vi "Get Instance Lookup.vi"(8 "error in (no error)":errorcluster, 10 "Create If Not Exist (T)":bool=TRUE, 11 "WebSocket In":refnum<class "Websocket.lvclass">) -> (0 "error out":errorcluster, 1 "NewObjectCreated":bool, 2 "DVRRefOut":refnum<data-value>, 3 "WebSocket Out":refnum<class "Websocket.lvclass">, 5 "ObjectQueueName":string caption="This queue name could be used to destroy\nthe named queue that is used to hold the\nreference in the clean up.")   [LabVIEW 2015]
uses:
  Websocket.lvclass
  Object Attributes.ctl
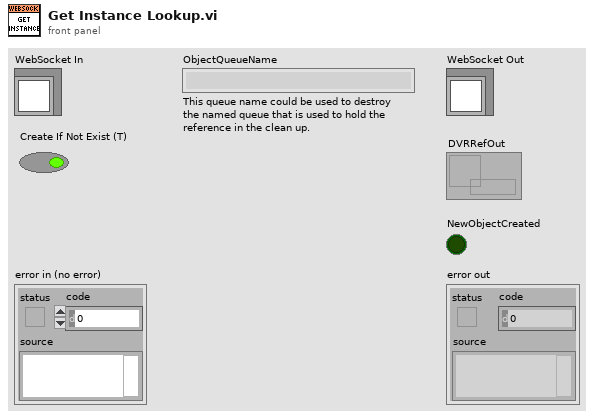
[diagram p1: front panel]
types:
  T1 = enum16{"Create or look up existing", "Look up existing"}
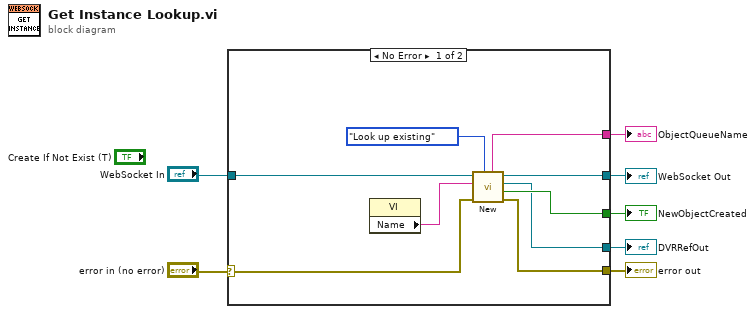
[diagram p0: block diagram]
diagram:
  n1 = case shown="No Error" "error in (no error)" {
    selector: "error in (no error)" -> [w15 w18]
    tunnel: [w16 w17] -> w7
    tunnel: [w14 w18] -> w5
    tunnel: "WebSocket In" -> [w12 w17]
    tunnel: [w11 _] -> w3
    tunnel: [w10 _] -> w2
    tunnel: [w8 _] -> w1
    frame No Error {
      n2 = property class="VI"() -> ("Name"=w13:string)  [unwired: 2 in, 2 out]
      n3 = call "New.vi"("CreateMethod(Create or look up existing)"=T1."Look up existing", "error in (no error)"=w15, "Object name"=w13, "Websocket In"=w12) -> ("error out"=w14:errorcluster, "NewObjectCreated"=w11:bool, "DVRRefOut"=w10:refnum<data-value>, "Websocket Out"=w16:refnum<class "Websocket.lvclass">, "ObjectQueueName"=w8:string)  [unwired: 3 in]
    }
    frame Error {
    }
  }
  "WebSocket Out" <- w7
  "error out" <- w5
  "NewObjectCreated" <- w3
  "DVRRefOut" <- w2
  "ObjectQueueName" <- w1
